vi "Algorithm.vi"(6 "IA State Input":T1={"our_robots"=[], "enemy_robots"=[], "balls"=[], "geometry"={"line_width"=0, "field_length"=0, "field_width"=0, "boundary_width"=0, "referee_width"=0, "goal_width"=0, "goal_depth"=0, "goal_wall_width"=0, "center_circle_radius"=0, "defense_radius"=0, "defense_stretch"=0, "free_kick_from_defense_dist"=0, "penalty_spot_from_field_line_dist"=0, "penalty_line_from_spot_dist"=0}, "IA Judge"={"stage"="", "command"="", "our_goalie_id"=0.0, "enemy_goalie_id"=0.0, "command enum"=enum."Halt", "Time"=enum."Azul"}, "Received Timestamp"=timestamp(0 s since 1904-01-01), "Events"={"Touch"=FALSE, "Ball out"=FALSE, "id touch"=0.0, "Ball out of \nVision"=FALSE, "Ball inside \nGoalie area"=FALSE, "Robot not responding"=FALSE, "Robots responding status"=[1.0, 1.0, 1.0, 1.0, 1.0, 1.0], "Enemy Ball \nPossession"=FALSE, "Pass State"=FALSE, "id end of pass"=0.0, "Kick"=FALSE, "Id ini Possession"=0.0, "Ball Possesion"=FALSE, "Id Possesion"=0.0}}, 7 "GridParameter":dbl=100.0, 8 "Ygoal":dbl format="%#_13g", 9 "Xgoal":dbl format="%#_13g", 10 "Ystart":dbl format="%#_13g", 11 "Xstart":dbl format="%#_13g") -> (2 "path":dbl[][](array[numeric]))   [LabVIEW 2017]
uses:
  elementGrid.ctl
  Core/AI Input.ctl
  Core/AI Robot.ctl
  Intel/Functions Enum.ctl
  Intel/AttackerStates.ctl
  RRT/PathDests.ctl
  RRT/PathDest.ctl
  Core/AI Ball.ctl
  Core/Field Size.ctl
  Core/AI Judge.ctl
  Intel/Command Enum.ctl
  Util/Events/Events.ctl
  AdvancedDataStructures/ClassBased/Applications/PriorityQueue/PriorityQueue/PriorityQueue.lvclass
  C:/Users/Rebeca/Documents/Rebeca/Roboime/SSLView/Path Planning/AdvancedDataStructures/ClassBased/LinkedList/LinkedList.lvclass
  AdvancedDataStructures/ClassBased/LinkedList/LinkedList.lvclass
  AdvancedDataStructures/ClassBased/Applications/PriorityQueue/PriorityQueue.lvlib
panel:
  out "reversed path":dbl[][](array[numeric])
  out "element":T12
  in  "dy":dbl[](array[numeric])=[1.0, -1.0, 0.0, 0.0, 1.0, -1.0, 1.0, -1.0]
  in  "dx":dbl[](array[numeric])=[0.0, 0.0, 1.0, -1.0, 1.0, 1.0, -1.0, -1.0]
  out "size":i32
  in  "Nó goal":dbl[](array[numeric])
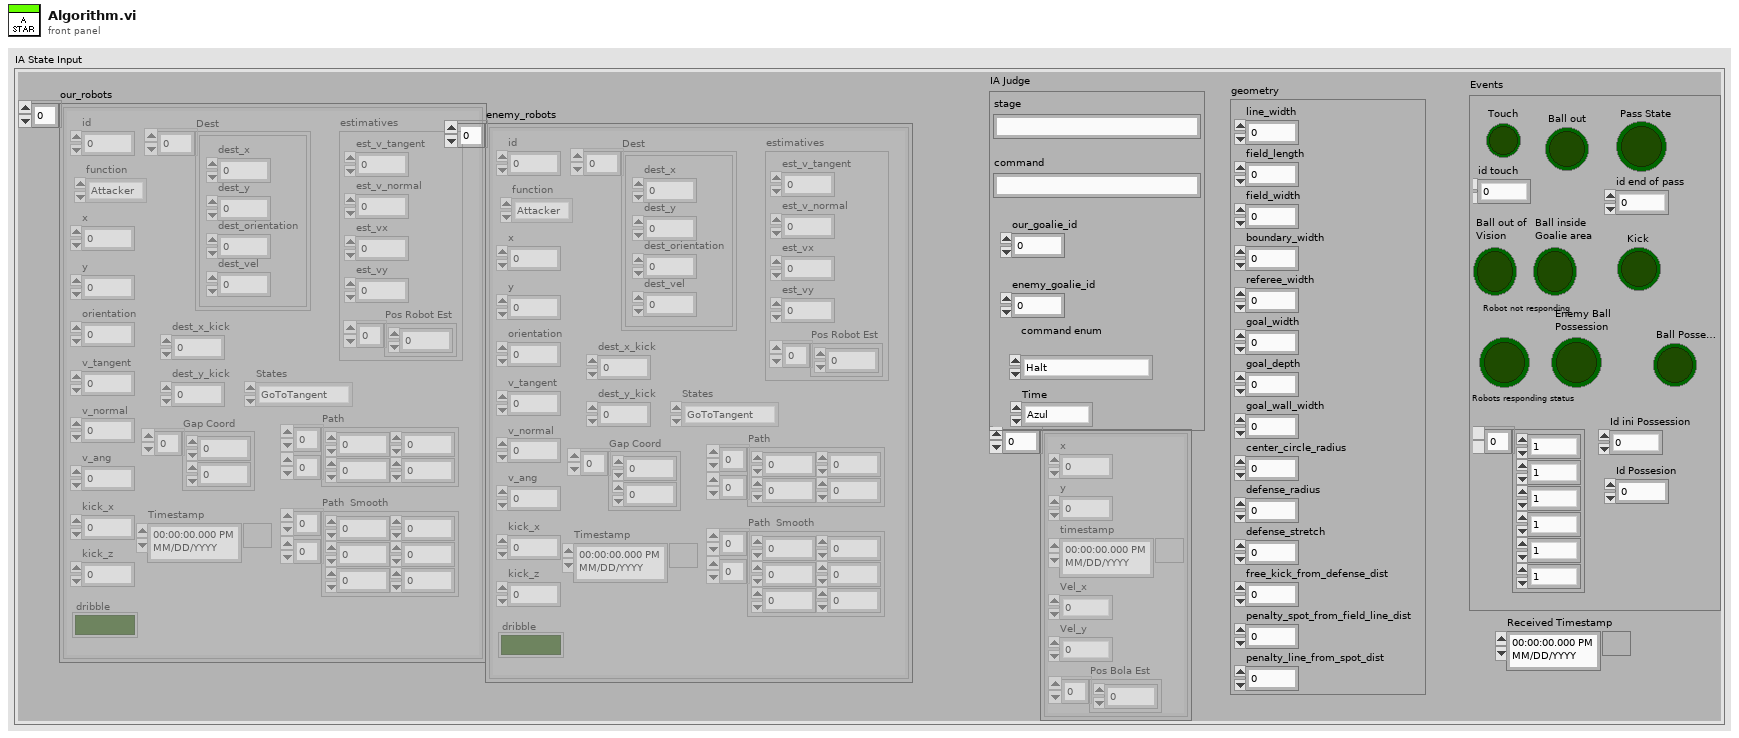
[diagram p1: front panel]
types:
  T1 = typedef "AI Input.ctl" = cluster{"our_robots":T2[], "enemy_robots":T2[], "balls":T7[], "geometry":T8, "IA Judge":T9, "Received Timestamp":timestamp, "Events":T11}
  T2 = typedef "AI Robot.ctl" = cluster{"id":u32, "function":T3, "x":dbl, "y":dbl, "orientation":dbl, "v_tangent":dbl, "v_normal":dbl, "v_ang":dbl, "kick_x":dbl, "kick_z":dbl, "dribble":bool, "Timestamp":timestamp, "estimatives":cluster{"est_v_tangent":dbl, "est_v_normal":dbl, "est_vx":dbl, "est_vy":dbl, "Pos Robot Est":dbl[]}, "dest_x_kick":dbl, "dest_y_kick":dbl, "Gap Coord":dbl[], "States":T4, "Path ":dbl[][], "Path  Smooth":dbl[][], "Dest":T5}
  T3 = typedef "Functions Enum.ctl" = enum16{"Attacker", "Goalie", "Defender", "Striker", "Goto 0", "Dummy", "Kicker", "ZigZag"}
  T4 = typedef "AttackerStates.ctl" = enum16{"Pass", "GoToTangent", "BallGetting", "GoToKick", ""}
  T5 = typedef "PathDests.ctl" = T6[]
  T6 = typedef "PathDest.ctl" = cluster{"dest_x":dbl, "dest_y":dbl, "dest_orientation":dbl, "dest_vel":dbl}
  T7 = typedef "AI Ball.ctl" = cluster{"x":dbl, "y":dbl, "timestamp":timestamp, "Vel_x":dbl, "Vel_y":dbl, "Pos Bola Est":dbl[]}
  T8 = typedef "Field Size.ctl" = cluster{"line_width":u32, "field_length":u32, "field_width":u32, "boundary_width":u32, "referee_width":u32, "goal_width":u32, "goal_depth":u32, "goal_wall_width":u32, "center_circle_radius":u32, "defense_radius":u32, "defense_stretch":u32, "free_kick_from_defense_dist":u32, "penalty_spot_from_field_line_dist":u32, "penalty_line_from_spot_dist":u32}
  T9 = typedef "AI Judge.ctl" = cluster{"stage":string, "command":string, "our_goalie_id":dbl, "enemy_goalie_id":dbl, "command enum":T10, "Time":enum16{"Azul", "Amarelo"}}
  T10 = typedef "Command Enum.ctl" = enum16{"Halt", "Stop", "Force Start", "PKA Normal Start", "Prepare Kickoff Ally", "PKE Normal Start", "Prepare Kickoff Enemy", "Prepare Penalty Ally", "PPA Normal Start", "Prepare Penalty Enemy", "PPE Normal Start", "Direct Free Enemy", "Direct Free Ally", "Indirect Free Enemy", "Indirect Free Ally", "Timeout Enemy", "Timeout Ally", "Goal Enemy", "Goal Ally", "Ball Placement Enemy", "Ball Placement Ally", "Normal Half Time", "Extra Time Break", "Extra Half Time", "None", "Post Game"}
  T11 = typedef "Events.ctl" = cluster{"Touch":bool, "Ball out":bool, "id touch":dbl, "Ball out of \nVision":bool, "Ball inside \nGoalie area":bool, "Robot not responding":bool, "Robots responding status":dbl[], "Enemy Ball \nPossession":bool, "Pass State":bool, "id end of pass":dbl, "Kick":bool, "Id ini Possession":dbl, "Ball Possesion":bool, "Id Possesion":dbl}
  T12 = typedef "elementGrid.ctl" = cluster{"id":dbl, "G":dbl, "H":dbl, "F":dbl, "x pai":dbl, "y pai":dbl}
  T13 = typedef "grid.ctl" = T12[][]
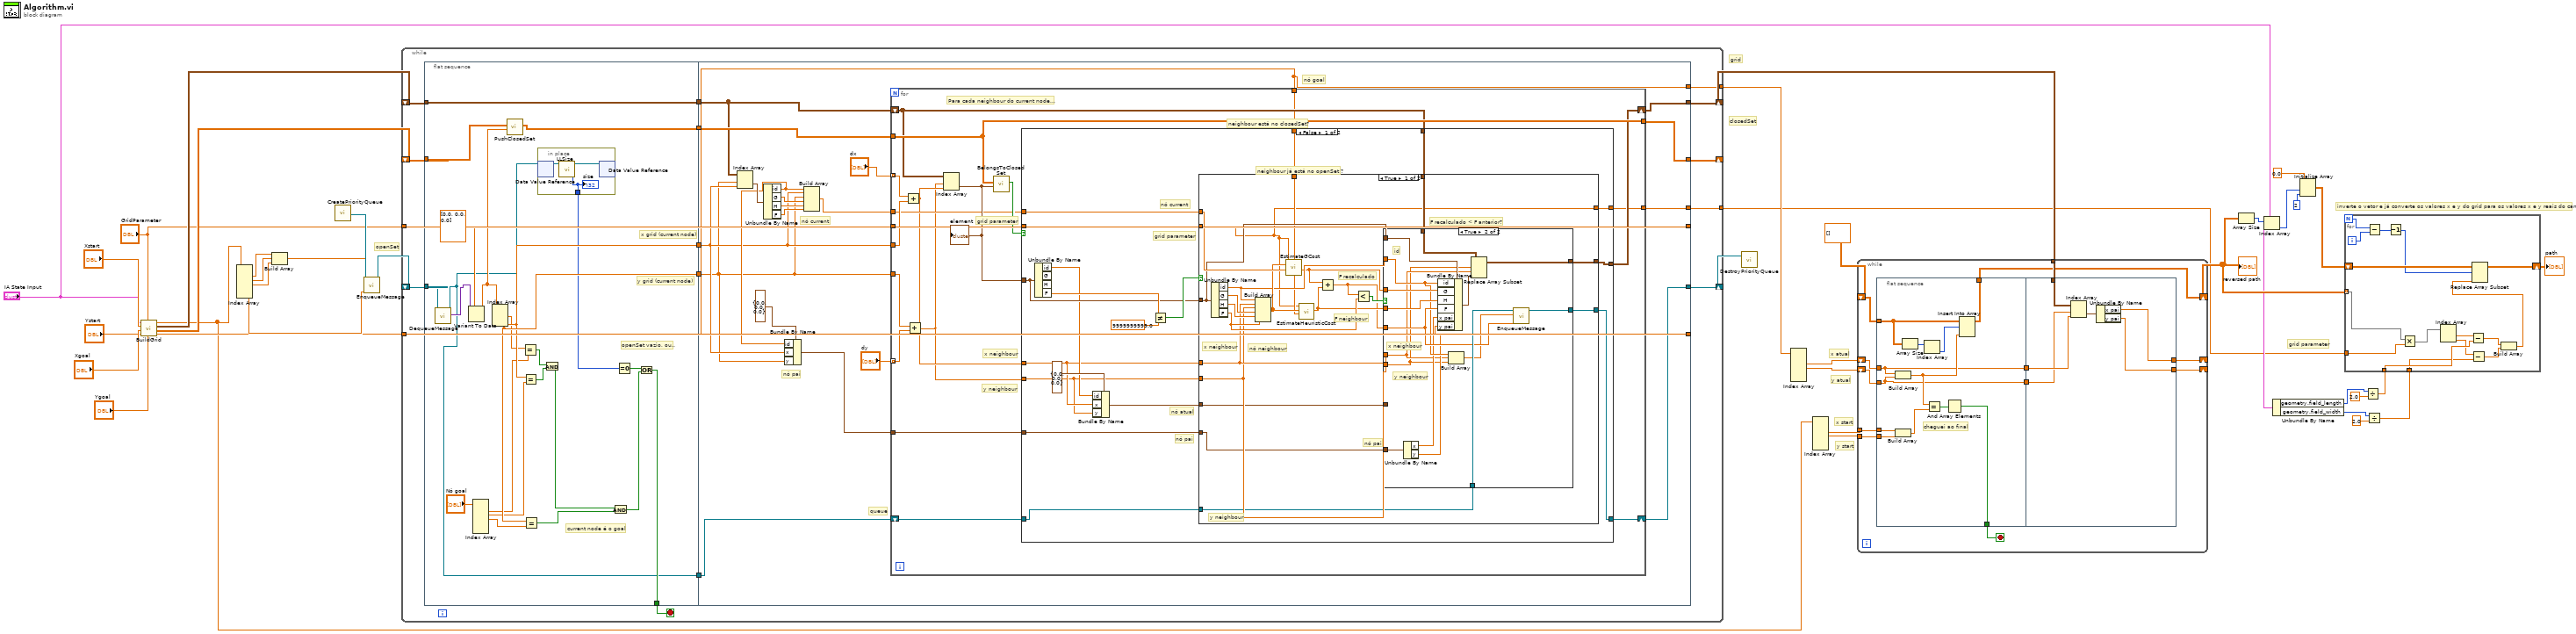
[diagram p0: block diagram]
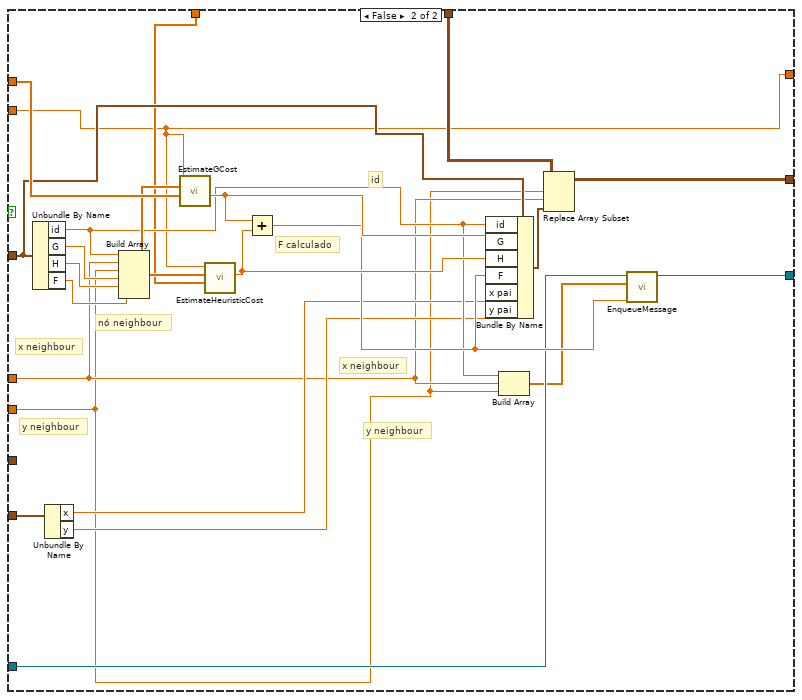
[diagram p3: hidden frame]
diagram:
  # "grid parameter"
  # "inverte o vetor e já converte os valores x e y do grid para os valores x e y reais do campo"
  # "y atual"
  # "x atual"
  # "y start"
  # "x start"
  # "closedSet"
  # "grid"
  # "openSet"
  n1 = call "BuildGrid.vi"("Ygoal"="Ygoal", "GridParameter"="GridParameter", "Ystart"="Ystart", "Xgoal"="Xgoal", "Xstart"="Xstart", "IA State Input"="IA State Input") -> ("Nó goal"=w6:dbl[], "ClosedSet out"=w29:dbl[][], "grid out"=w30:T13, "Nó start"=w4:dbl[])  [unwired: 2 in]
  n2 = Index Array(array=w4) -> (element #1=w28:dbl, element #2=w27:dbl, element #3=w34:dbl, element #6=w32:dbl)  [unwired: 6 in, 2 out]
  n3 = Build Array(w28, w27, w34) -> (w33:dbl[])
  n4 = call "CreatePriorityQueue.vi"() -> ("PriorityQueue"=w35:refnum<data-value>)  [unwired: 10 in, 1 out]
  n5 = call "EnqueueMessage.vi"("Priority"=w32, "message"=w33, "queue in"=w35) -> ("queue out"=w31:refnum<data-value>)  [unwired: 7 in, 1 out]
  n6 = while {
    shift-right: [w45] -> w26
    shift-left: w31 -> [w55]
    shift-right: [w44] -> w20
    shift-left: w30 -> [w48]
    shift-right: [w47] -> _
    shift-left: w29 -> [w54]
    tunnel: w6 -> [w43]
    tunnel: [w42] -> w5
    tunnel: "GridParameter" -> [w41]
    tunnel: [w40] -> w1
    stop <- w53 stop-if-true
    n7 = flat-sequence {
      tunnel: w55 -> [w78]
      tunnel: w54 -> [w75]
      tunnel: [w62] -> w53
      tunnel: [w77] -> w52
      tunnel: [w76] -> w51
      tunnel: [w58] -> w50
      tunnel: [w57] -> w49
      tunnel: w48 -> [w57]
      tunnel: [w56] -> w46
      tunnel: w52 -> [w85]
      tunnel: w51 -> [w86]
      tunnel: w50 -> [w100]
      tunnel: w49 -> [w96]
      tunnel: [w99] -> w47
      tunnel: w46 -> [w98]
      tunnel: [w97] -> w45
      tunnel: [w90] -> w44
      tunnel: w43 -> [w84]
      tunnel: [w84] -> w42
      tunnel: w41 -> [w83]
      tunnel: [w82] -> w40
      frame #0 {
        # "y grid (current node)"
        # "x grid (current node)"
        # "current node é o goal"
        # "openSet vazio, ou.."
        n8 = call "DequeueMessage.vi"("queue in"=w78) -> ("message"=w61:variant, "queue out"=w56:refnum<data-value>)  [unwired: 7 in, 2 out]
        n9 = Variant To Data(type=dbl[] [0.0, 0.0, 0.0] ("New Node"), Variant=w61) -> (data=w63:dbl[])  [unwired: 1 in, 1 out]
        n10 = Index Array(array="Nó goal") -> (element #1=w72:dbl, element #2=w71:dbl, element #3=w70:dbl)  [unwired: 6 in, 3 out]
        n11 = Index Array(array=w63) -> (element #1=w64:dbl, element #2=w76:dbl, element #3=w77:dbl)  [unwired: 3 in]
        n12 = call "PushClosedSet.vi"("Novo nó"=w63, "ClosedSet"=w75) -> ("NewClosedSet"=w58:dbl[][])  [unwired: 9 in]
        n13 = Equal?(x=w64, y=w72) -> (x = y?=w69:bool)
        n14 = Equal?(x=w76, y=w71) -> (x = y?=w68:bool)
        n15 = Equal?(x=w77, y=w70) -> (x = y?=w66:bool)
        n16 = in-place {
          in-place-border: [w79] -> w60
          n17 = in-place-dvr #1(w56) -> (w81:refnum<class "PriorityQueue.lvclass">)  [unwired: 1 out]
          n18 = call "LLSize.vi"("LinkedList in"=w81) -> ("size"=w79:i32, "LinkedList out"=w80:refnum<class "PriorityQueue.lvclass">)  [unwired: 8 in, 1 out]
          "size" <- w79
          n19 = in-place-dvr #1(w80) -> ()  [unwired: 2 out]
        }
        n20 = And(x=w69, y=w68) -> (x .and. y?=w67:bool)
        n21 = And(x=w67, y=w66) -> (x .and. y?=w65:bool)
        n22 = Equal To 0?(x=w60) -> (x = 0?=w59:bool)
        n23 = Or(x=w59, y=w65) -> (x .or. y?=w62:bool)
      }
      frame #1 {
        # "nó goal"
        # "nó pai"
        # "nó current"
        # "queue"
        n24 = Index Array(array=w96, index (row)=w85, index (col)=w86) -> (element=w95:T12)
        n25 = Unbundle By Name(w95) -> ("id"=w88:dbl, "G"=w94:dbl, "H"=w93:dbl, "F"=w92:dbl)
        n26 = Bundle By Name(cluster=cluster{"id":dbl, "x":dbl, "y":dbl} {"id"=0.0, "x"=0.0, "y"=0.0} ("nó atual"), "id"=w88, "x"=w86, "y"=w85) -> (w87:cluster{"id":dbl, "x":dbl, "y":dbl})
        n27 = Build Array(w88, w86, w85, w94, w93, w92) -> (w91:dbl[])
        n28 = for {
          tunnel: "dx" -> [w120] mode=indexing
          tunnel: "dy" -> [w117] mode=indexing
          tunnel: w86 -> [w119]
          tunnel: w85 -> [w118]
          shift-right: [w109] -> w90
          shift-left: w96 -> [w110]
          tunnel: w100 -> [w115]
          tunnel: [w115] -> w99
          shift-right: [w112] -> w97
          shift-left: w98 -> [w114]
          tunnel: w91 -> [w111]
          tunnel: w87 -> [w108]
          tunnel: w84 -> [w105]
          tunnel: w83 -> [w104]
          tunnel: [w103] -> w82
          # "grid parameter"
          # "y neighbour"
          # "x neighbour"
          # "neighbour está no closedSet?"
          # "Para cada neighbour do current node..."
          n29 = Add(x=w120, y=w119) -> (x+y=w107:dbl)
          n30 = Add(x=w118, y=w117) -> (x+y=w106:dbl)
          n31 = Index Array(array=w110, index (row)=w106, index (col)=w107) -> (element=w113:T12)
          "element" <- w113
          n32 = call "BelongsToClosedSet.vi"("neighbour"=w113, "ClosedSet in"=w115) -> ("belongs_to_closedSet"=w116:bool)  [unwired: 9 in]
          n33 = case shown="False" w116 {
            tunnel: w114 -> [w132 w203]
            tunnel: [w131 w203] -> w112
            tunnel: w113 -> [w130 _]
            tunnel: w107 -> [w126 _]
            tunnel: w106 -> [w125 _]
            tunnel: w111 -> [w135 _]
            tunnel: w110 -> [w134 w202]
            tunnel: [w133 w202] -> w109
            tunnel: w108 -> [w129 _]
            tunnel: w105 -> [w123 _]
            tunnel: w104 -> [w122 w201]
            tunnel: [w121 w201] -> w103
            frame False {
              # "grid parameter"
              # "nó atual"
              # "nó pai"
              # "nó current"
              # "neighbour já está no openSet ?"
              n34 = Unbundle By Name(w130) -> ("id"=w127:dbl, "F"=w138:dbl)  [unwired: 2 out]
              n35 = Bundle By Name(cluster=cluster{"id":dbl, "x":dbl, "y":dbl} {"id"=0.0, "x"=0.0, "y"=0.0} ("nó atual"), "id"=w127, "x"=w126, "y"=w125) -> (w124:cluster{"id":dbl, "x":dbl, "y":dbl})
              n36 = Not Equal?(x=w138, y=9999999999.0) -> (x != y?=w136:bool)
              n37 = case shown="True" w136 {
                tunnel: w130 -> [w146 w191]
                tunnel: w126 -> [w152 w181]
                tunnel: w125 -> [w151 w180]
                tunnel: w135 -> [w157 w198]
                tunnel: w134 -> [w153 w195]
                tunnel: [w145 w190] -> w133
                tunnel: w132 -> [w144 w189]
                tunnel: [w143 w188] -> w131
                tunnel: w129 -> [w141 w184]
                tunnel: w124 -> [w142 _]
                tunnel: w123 -> [w140 w179]
                tunnel: w122 -> [w139 w178]
                tunnel: [w139 w178] -> w121
                frame True {
                  # "nó pai"
                  # "F recalculado < F anterior?"
                  # "F neighbour"
                  # "F recalculado"
                  # "nó neighbour"
                  # "y neighbour"
                  # "x neighbour"
                  n38 = Unbundle By Name(w146) -> ("id"=w150:dbl, "G"=w159:dbl, "H"=w158:dbl, "F"=w155:dbl)
                  n39 = Build Array(w150, w152, w151, w159, w158, w155) -> (w156:dbl[])
                  n40 = call "EstimateGCost.vi"("Nó pai"=w157, "Nó atual"=w156, "GridParameter"=w139) -> ("G_Cost"=w149:dbl)  [unwired: 8 in]
                  n41 = call "EstimateHeuristicCost.vi"("Goal"=w140, "Nó atual"=w156, "GridParameter"=w139) -> ("Heuristic"=w148:dbl)  [unwired: 8 in]
                  n42 = Add(x=w149, y=w148) -> (x+y=w147:dbl)
                  n43 = Less?(x=w147, y=w155) -> (x < y?=w154:bool)
                  n44 = case shown="True" w154 {
                    tunnel: w153 -> [w160 w177]
                    tunnel: w152 -> [_ w163]
                    tunnel: w151 -> [_ w162]
                    tunnel: w150 -> [_ w169]
                    tunnel: w149 -> [_ w176]
                    tunnel: w148 -> [_ w175]
                    tunnel: w147 -> [_ w170]
                    tunnel: w146 -> [_ w174]
                    tunnel: [w160 w172] -> w145
                    tunnel: w144 -> [w161 w171]
                    tunnel: [w161 w167] -> w143
                    tunnel: w142 -> [_ _]
                    tunnel: w141 -> [_ w166]
                    frame False {
                    }
                    frame True {
                      # "id"
                      # "y neighbour"
                      # "x neighbour"
                      n45 = Unbundle By Name(w166) -> ("x"=w165:dbl, "y"=w164:dbl)
                      n46 = Bundle By Name(cluster=w174, "id"=w169, "G"=w176, "H"=w175, "F"=w170, "x pai"=w165, "y pai"=w164) -> (w173:T12)
                      n47 = Build Array(w169, w163, w162) -> (w168:dbl[])
                      n48 = Replace Array Subset(array=w177, new element=w173, index (row)=w162, index (col)=w163) -> (w172:T13)
                      n49 = call "EnqueueMessage.vi"("Priority"=w170, "message"=w168, "queue in"=w171) -> ("queue out"=w167:refnum<data-value>)  [unwired: 7 in, 1 out]
                    }
                  }
                }
                frame False {
                  # "F calculado"
                  # "id"
                  # "y neighbour"
                  # "x neighbour"
                  # "nó neighbour"
                  # "y neighbour"
                  # "x neighbour"
                  n50 = Unbundle By Name(w191) -> ("id"=w185:dbl, "G"=w200:dbl, "H"=w199:dbl, "F"=w196:dbl)
                  n51 = Unbundle By Name(w184) -> ("x"=w183:dbl, "y"=w182:dbl)
                  n52 = Build Array(w185, w181, w180, w200, w199, w196) -> (w197:dbl[])
                  n53 = call "EstimateGCost.vi"("Nó pai"=w198, "Nó atual"=w197, "GridParameter"=w178) -> ("G_Cost"=w194:dbl)  [unwired: 8 in]
                  n54 = call "EstimateHeuristicCost.vi"("Goal"=w179, "Nó atual"=w197, "GridParameter"=w178) -> ("Heuristic"=w193:dbl)  [unwired: 8 in]
                  n55 = Add(x=w194, y=w193) -> (x+y=w192:dbl)
                  n56 = Bundle By Name(cluster=w191, "id"=w185, "G"=w194, "H"=w193, "F"=w192, "x pai"=w183, "y pai"=w182) -> (w187:T12)
                  n57 = Build Array(w185, w181, w180) -> (w186:dbl[])
                  n58 = Replace Array Subset(array=w195, new element=w187, index (row)=w180, index (col)=w181) -> (w190:T13)
                  n59 = call "EnqueueMessage.vi"("Priority"=w192, "message"=w186, "queue in"=w189) -> ("queue out"=w188:refnum<data-value>)  [unwired: 7 in, 1 out]
                }
              }
            }
            frame True {
            }
          }
        }
      }
    }
  }
  n60 = call "DestroyPriorityQueue.vi"("Queue"=w26) -> ()  [unwired: 10 in, 1 out]
  n61 = Index Array(array=w5) -> (element #2=w23:dbl, element #3=w22:dbl)  [unwired: 6 in, 4 out]
  n62 = Index Array(array=w4) -> (element #2=w25:dbl, element #3=w24:dbl)  [unwired: 6 in, 4 out]
  n63 = while {
    tunnel: w25 -> [w212]
    tunnel: w24 -> [w211]
    shift-right: [w206] -> _
    shift-left: w23 -> [w214]
    shift-right: [w205] -> _
    shift-left: w22 -> [w213]
    shift-right: [w204] -> w17
    shift-left: dbl[][] [] ("Path 2") -> [w215]
    tunnel: w20 -> [w209]
    stop <- w210 stop-if-true
    n64 = flat-sequence {
      tunnel: w215 -> [w227]
      tunnel: w214 -> [w218]
      tunnel: w213 -> [w217]
      tunnel: w212 -> [w224]
      tunnel: w211 -> [w223]
      tunnel: [w219] -> w210
      tunnel: [w218] -> w208
      tunnel: [w217] -> w207
      tunnel: [w216] -> w204
      tunnel: w209 -> [w233]
      tunnel: w208 -> [w232]
      tunnel: w207 -> [w231]
      tunnel: [w229] -> w206
      tunnel: [w228] -> w205
      frame #0 {
        # "cheguei ao final"
        n65 = Build Array(w224, w223) -> (w221:dbl[])
        n66 = Build Array(w218, w217) -> (w222:dbl[])
        n67 = Array Size(array=w227) -> (size(s)=w226:i32[])
        n68 = Index Array(array=w226) -> (element=w225:i32)  [unwired: 1 in]
        n69 = Equal?(x=w222, y=w221) -> (x = y?=w220:bool[])
        n70 = And Array Elements(Boolean array=w220) -> (logical AND=w219:bool)
        n71 = Insert Into Array(array=w227, index (row)=w225, new element=w222) -> (w216:dbl[][])  [unwired: 1 in]
      }
      frame #1 {
        n72 = Index Array(array=w233, index (row)=w231, index (col)=w232) -> (element=w230:T12)
        n73 = Unbundle By Name(w230) -> ("x pai"=w229:dbl, "y pai"=w228:dbl)
      }
    }
  }
  "reversed path" <- w17
  n74 = Array Size(array=w17) -> (size(s)=w16:i32[])
  n75 = Index Array(array=w16) -> (element=w15:i32)  [unwired: 1 in]
  n76 = Unbundle By Name("IA State Input") -> ("geometry.field_length"=w9:u32, "geometry.field_width"=w10:u32)
  n77 = Initialize Array(0.0 ("element"), w15, 2 ("dimension size")) -> (w14:dbl[][])
  n78 = Divide(x=w9, y=2.0) -> (x/y=w8:dbl)
  n79 = Divide(x=w10, y=2.0) -> (x/y=w7:dbl)
  n80 = for {
    N -> [w248]
    tunnel: w17 -> [w243] mode=indexing
    shift-right: [w244] -> w13
    shift-left: w14 -> [w249]
    tunnel: w8 -> [w240]
    tunnel: w7 -> [w238]
    tunnel: w1 -> [w234]
    i -> [w247]
    n81 = Subtract(x=w248, y=w247) -> (x-y=w246:i32)
    n82 = Decrement(x=w246) -> (x-1=w245:i32)
    n83 = Multiply(x=w243, y=w234) -> (x*y=w242:dbl[])
    n84 = Index Array(array=w242) -> (element #1=w241:dbl, element #2=w239:dbl)  [unwired: 2 in]
    n85 = Subtract(x=w241, y=w240) -> (x-y=w237:dbl)
    n86 = Subtract(x=w239, y=w238) -> (x-y=w236:dbl)
    n87 = Build Array(w237, w236) -> (w235:dbl[])
    n88 = Replace Array Subset(array=w249, new element=w235, index (row)=w245) -> (w244:dbl[][])  [unwired: 1 in]
  }
  "path" <- w13
